vi "Save Load Gear Mech Settings.vi"(8 "error in":errorcluster, 10 "Gear Mech Settings (in)":T1={"Out Speed"=-0.5, "In Speed"=0.5, "Up Position"=560.0, "Down Position"=345.0, "Full Up Position"=600.0, "Gear PID"={"D"=0.01, "F"=0.0, "RR"=0.0, "IZ"=0.0, "P"=3.0, "I"=0.0}}, 11 "Save Load Info":T3) -> (0 "error out":errorcluster, 2 "Gear Mech Settings (out)":T1={"Out Speed"=-0.5, "In Speed"=0.5, "Up Position"=560.0, "Down Position"=345.0, "Full Up Position"=600.0, "Gear PID"={"D"=0.01, "F"=0.0, "RR"=0.0, "IZ"=0.0, "P"=3.0, "I"=0.0}}, 3 "Save Load Info (out)":T3)   [LabVIEW 2016]
uses:
  Load Save Info.ctl
  <vilib>/Utility/config.llb/Config Data RefNum.ctl
  Gear Mech Settings.ctl
  PID Settings.ctl
  <vilib>/Utility/config.llb/NI_LVConfig.lvlib
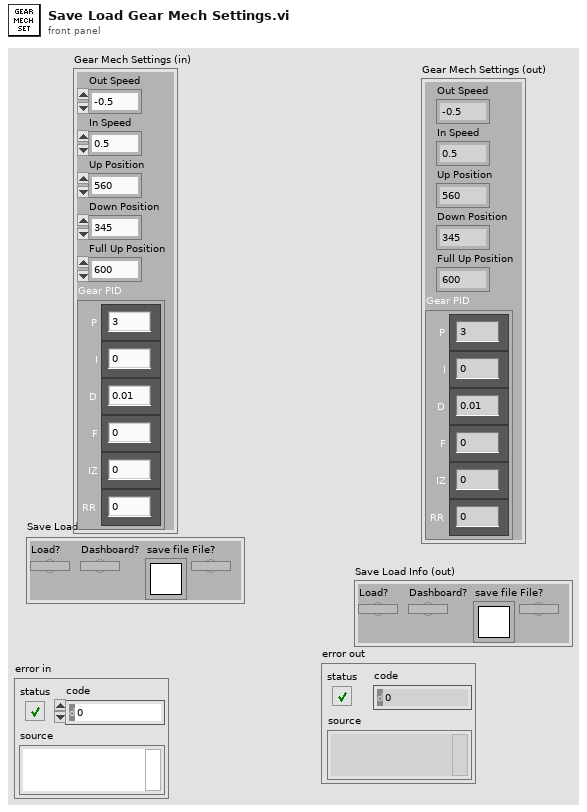
[diagram p1: front panel]
types:
  T1 = typedef "Gear Mech Settings.ctl" = cluster{"Out Speed":dbl, "In Speed":dbl, "Up Position":dbl, "Down Position":dbl, "Full Up Position":dbl, "Gear PID":T2}
  T2 = typedef "PID Settings.ctl" = cluster{"D":dbl, "F":dbl, "RR":dbl, "IZ":dbl, "P":dbl, "I":dbl}
  T3 = typedef "Load Save Info.ctl" = cluster{"Load?":bool, "Dashboard?":bool, "save file":T4, "File?":bool}
  T4 = typedef "NI_LVConfig.lvlib/Config Data RefNum.ctl" = refnum<k1>
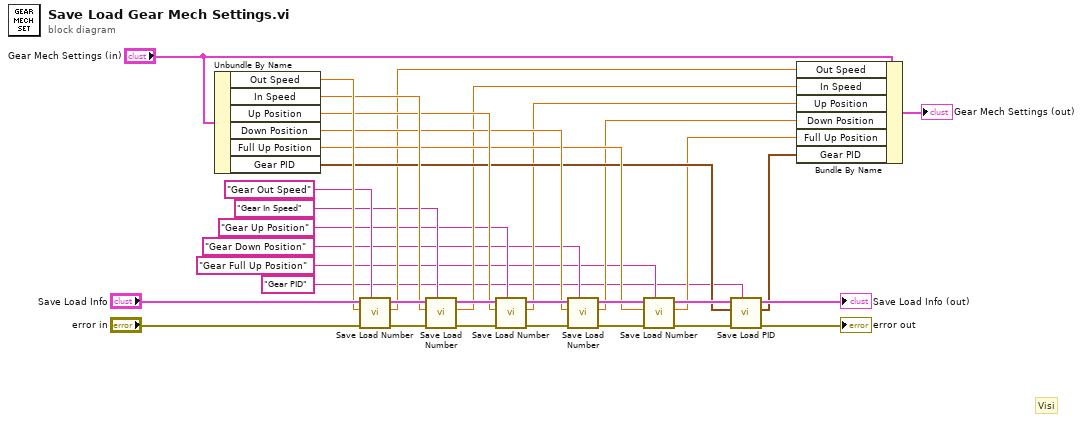
[diagram p0: block diagram]
diagram:
  # "Visi"
  n1 = Unbundle By Name("Gear Mech Settings (in)") -> ("Out Speed"=w19:dbl, "In Speed"=w18:dbl, "Up Position"=w17:dbl, "Down Position"=w16:dbl, "Full Up Position"=w15:dbl, "Gear PID"=w14:T2)
  n2 = call "Save Load Number.vi"("Name"="Gear Out Speed", "error in"="error in", "Num (in)"=w19, "Save Load Info (in)"="Save Load Info") -> ("error out"=w32:errorcluster, "Num (out)"=w12:dbl, "Save Load Info (out)"=w23:T3)  [unwired: 5 in]
  n3 = call "Save Load Number.vi"("Name"="Gear In Speed", "error in"=w32, "Num (in)"=w18, "Save Load Info (in)"=w23) -> ("error out"=w31:errorcluster, "Num (out)"=w11:dbl, "Save Load Info (out)"=w22:T3)  [unwired: 5 in]
  n4 = call "Save Load Number.vi"("Name"="Gear Up Position", "error in"=w31, "Num (in)"=w17, "Save Load Info (in)"=w22) -> ("error out"=w30:errorcluster, "Num (out)"=w10:dbl, "Save Load Info (out)"=w21:T3)  [unwired: 5 in]
  n5 = call "Save Load Number.vi"("Name"="Gear Down Position", "error in"=w30, "Num (in)"=w16, "Save Load Info (in)"=w21) -> ("error out"=w29:errorcluster, "Num (out)"=w9:dbl, "Save Load Info (out)"=w20:T3)  [unwired: 5 in]
  n6 = call "Save Load Number.vi"("Name"="Gear Full Up Position", "error in"=w29, "Num (in)"=w15, "Save Load Info (in)"=w20) -> ("error out"=w28:errorcluster, "Num (out)"=w8:dbl, "Save Load Info (out)"=w25:T3)  [unwired: 5 in]
  n7 = call "Save Load PID.vi"("Name"="Gear PID", "error in"=w28, "PID (in)"=w14, "Save Load Info (in)"=w25) -> ("error out"=→"error out":errorcluster, "PID (out)"=w7:T2, "Save Load Info (out)"=→"Save Load Info (out)":T3)  [unwired: 5 in]
  n8 = Bundle By Name(cluster="Gear Mech Settings (in)", "Out Speed"=w12, "In Speed"=w11, "Up Position"=w10, "Down Position"=w9, "Full Up Position"=w8, "Gear PID"=w7) -> (→"Gear Mech Settings (out)":T1)
